vi "main.vi"() -> ()   [LabVIEW 2016]
uses:
  Control 1.ctl
  Antenna.ctl
  Cable 1.ctl
  Cable 2.ctl
  Cable 3.ctl
  Attenuator.ctl
  Amplifier.ctl
  Limit.ctl
  Prescan Spec An Setting.ctl
  Frequency Range.ctl
panel:
  in  "Main":T1(tab)
  in  "Test Configuration":T2(tab)
  in  "Antenna":T3
  in  "Cable 1":T4
  in  "Cable 2":T5
  in  "Cable 3":T6
  in  "Amplifier":T7=enum."10K-2GHz ME813"
  in  "Attenuator":T8
  in  "Limit":T9
  in  "Start Frequecny (MHz)":dbl
  in  "Stop Frequecny (MHz)":dbl
  in  "Generate":bool
  in  "Frequency \nRange":T10
  in  "Prescan \nSpec An \nSetting":T11={"Reference Level (dBuV)"=107.0, "Attenuation (dB)"=10.0, "Step Size (KHz)"=90.0, "RBW (KHz)"=120.0, "VBW (KHz)"=300.0, "Dwell Time (ms)"=0.1, "Detector"=enum."Peak"}
  out "Table Control":string[][](table)
  in  "Prescan Accept":bool
  in  "Start Prescan":bool
  out "Prescan Plot":cluster{"xi used":dbl[], "yi":dbl[]}[](graph)
  in  "Final Accept":bool
  in  "Final Measurement":bool
  out "Equipment ID":string
  in  "VISA input":refnum<visa-resource-name>
  out "Current status":T12
  in  "Stop":bool
  in  "Generate Report":bool
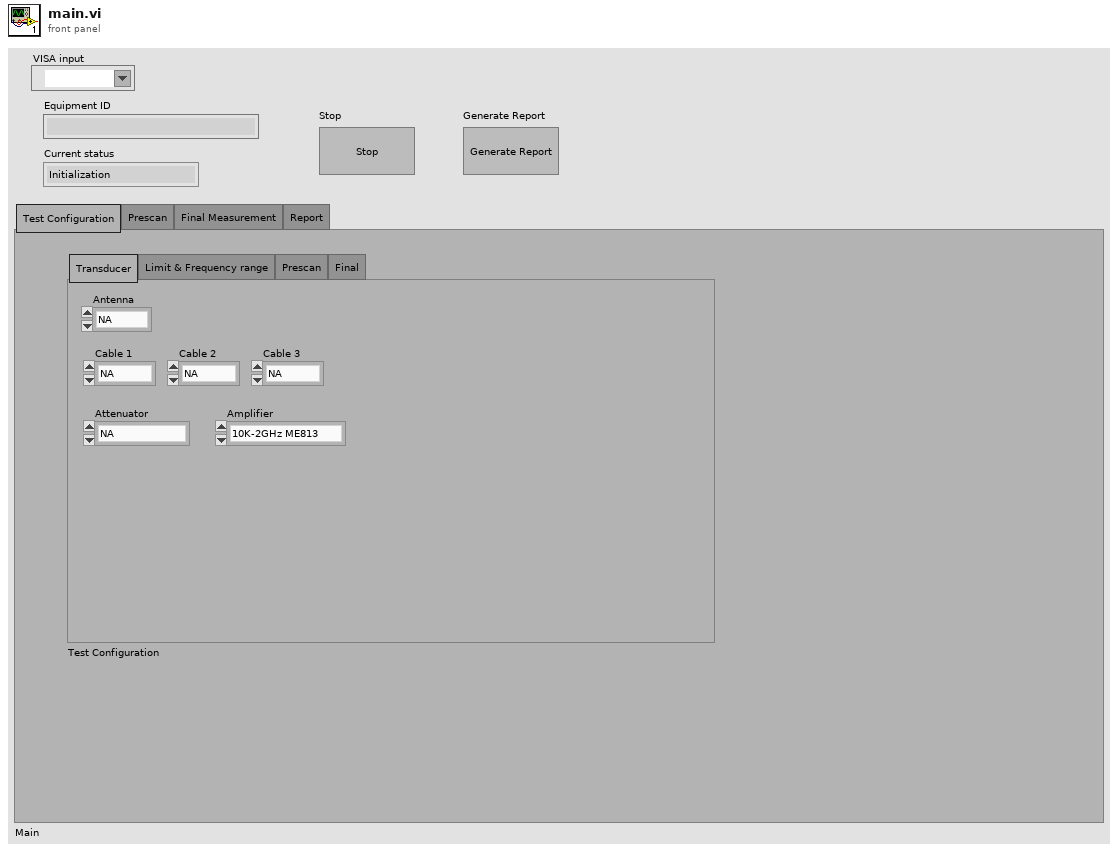
[diagram p1: front panel]
types:
  T1 = enum32{"Test Configuration", "Prescan", "Final Measurement", "Report"}
  T2 = enum32{"Transducer", "Limit & Frequency range", "Prescan", "Final"}
  T3 = typedef "Antenna.ctl" = enum16{"NA", "ME828 Biconical", "ME1284 Periodical"}
  T4 = typedef "Cable 1.ctl" = enum16{"NA", "ME1244", "ME1245", "ME1249"}
  T5 = typedef "Cable 2.ctl" = enum16{"NA", "ME1244", "ME1245", "ME1249"}
  T6 = typedef "Cable 3.ctl" = enum16{"NA", "ME1244", "ME1245", "ME1249"}
  T7 = typedef "Amplifier.ctl" = enum16{"NA", "10K-2GHz ME813", "500M-18GHz ME1241"}
  T8 = typedef "Attenuator.ctl" = enum16{"NA", "6dB-ME811"}
  T9 = typedef "Limit.ctl" = enum16{"NA", "CISPR32 ClassB @ 3m"}
  T10 = typedef "Frequency Range.ctl" = enum32{"20-300MHz", "300-1000MHz", "1-18GHz"}
  T11 = typedef "Prescan Spec An Setting.ctl" = cluster{"Reference Level (dBuV)":dbl, "Attenuation (dB)":dbl, "Step Size (KHz)":dbl, "RBW (KHz)":dbl, "VBW (KHz)":dbl, "Dwell Time (ms)":dbl, "Detector":enum16{"Peak", "CISPR Peak", "Mil Peak", "Quasi Peak", "Average"}}
  T12 = typedef "Control 1.ctl" = enum16{"Initialization", "IDLE (wait for event)", "Prescan test configuration", "Prescan", "Final test configuration", "Final measurement", "Report", "Stop"}
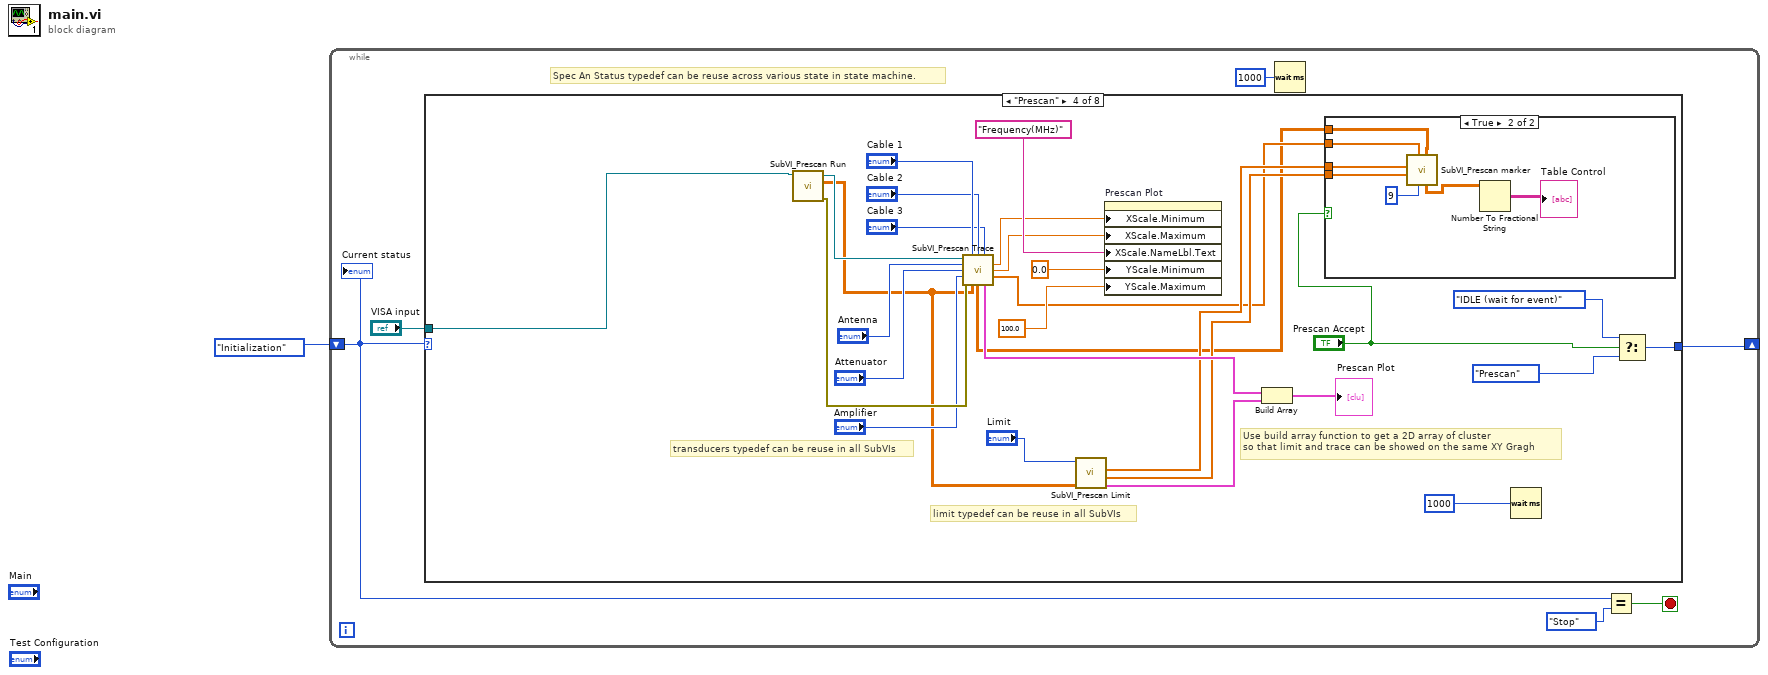
[diagram p0: block diagram]
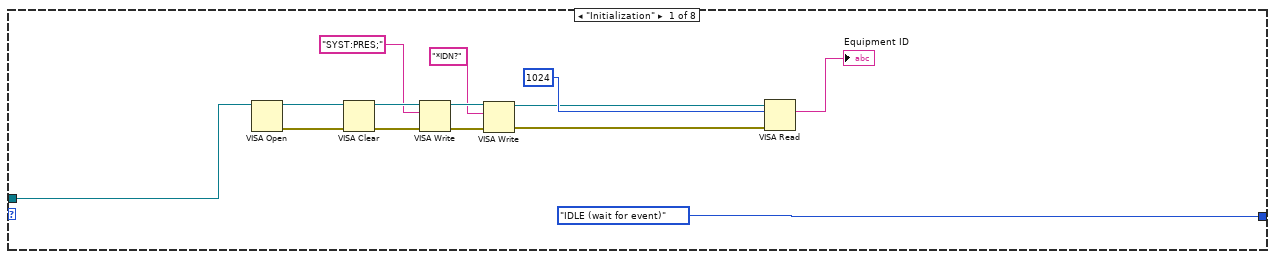
[diagram p2: hidden frame]
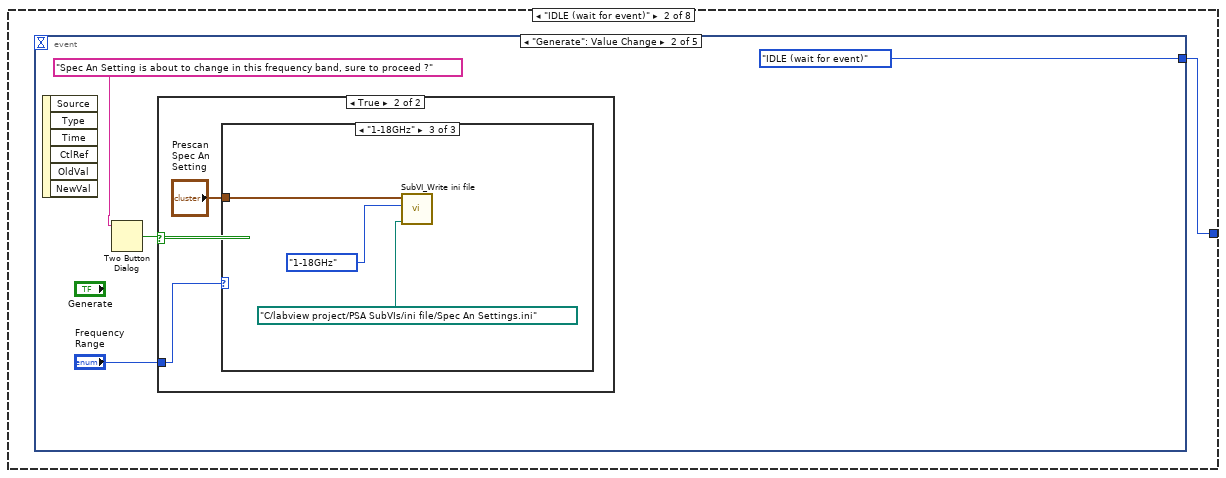
[diagram p3: hidden frame]
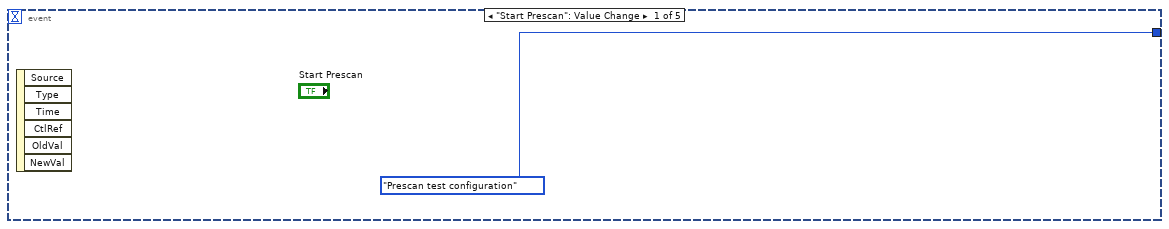
[diagram p4: hidden frame]
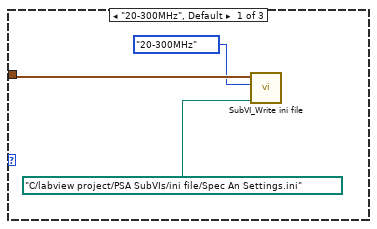
[diagram p6: hidden frame]
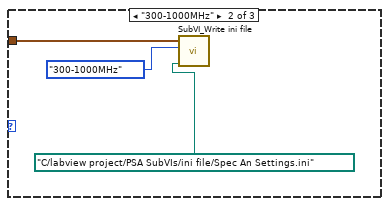
[diagram p7: hidden frame]
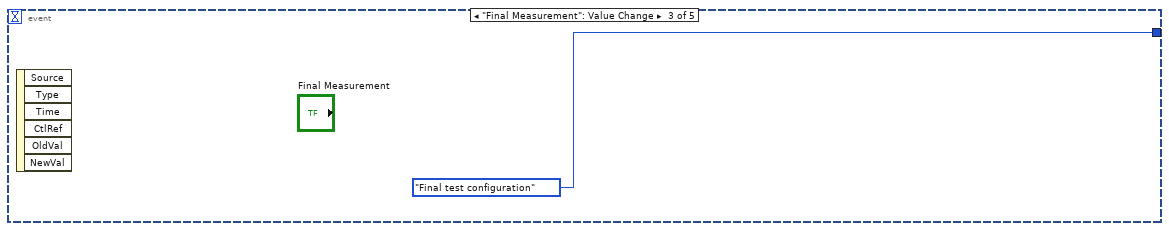
[diagram p8: hidden frame]
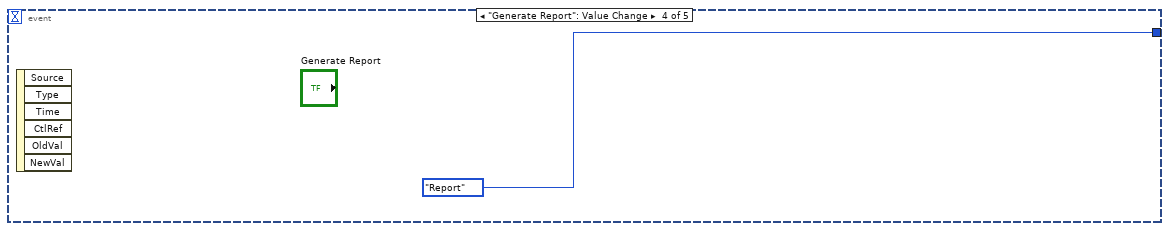
[diagram p9: hidden frame]
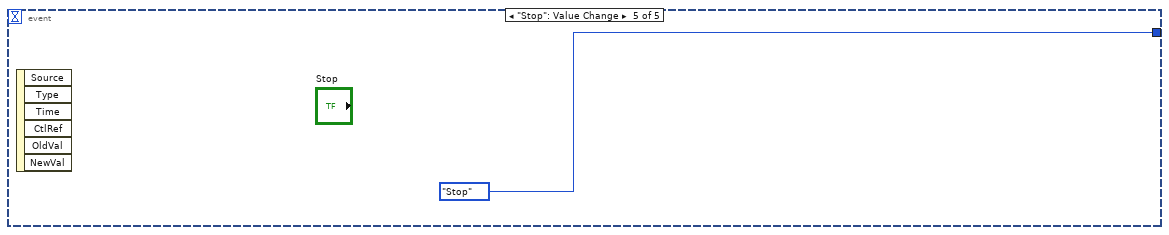
[diagram p10: hidden frame]
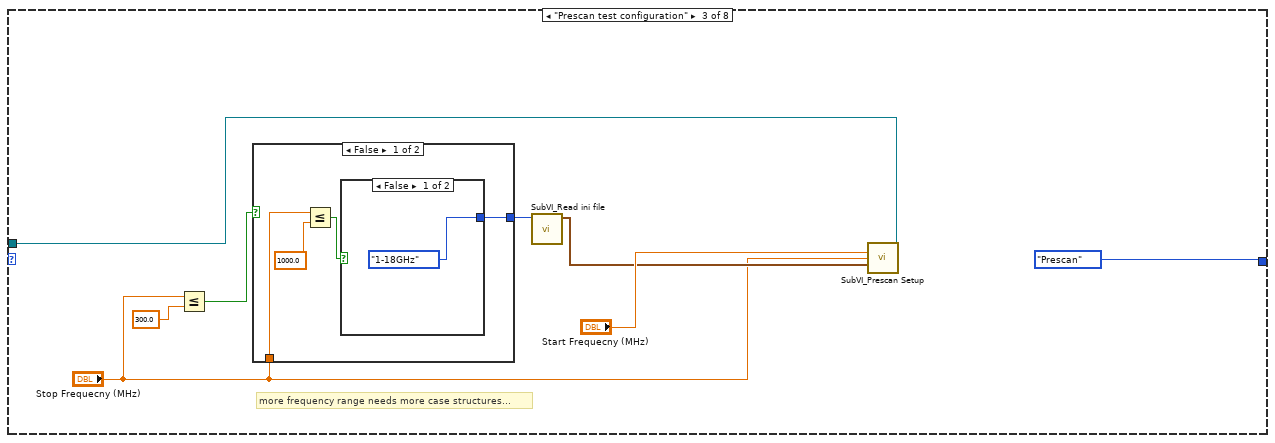
[diagram p11: hidden frame]
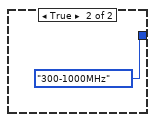
[diagram p12: hidden frame]
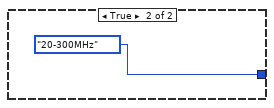
[diagram p13: hidden frame]
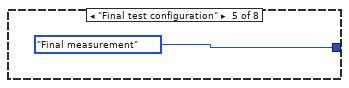
[diagram p15: hidden frame]
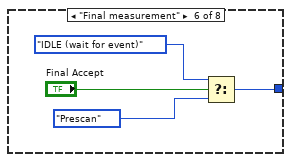
[diagram p16: hidden frame]
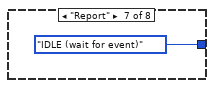
[diagram p17: hidden frame]
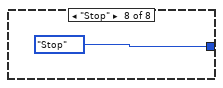
[diagram p18: hidden frame]
diagram:
  n1 = while {
    shift-right: [w6] -> _
    shift-left: Control_1."Initialization" -> [w2]
    stop <- w4 stop-if-true
    # "Spec An Status typedef can be reuse across various state in state machine."
    n2 = case shown="\"Prescan\"" w2 {
      tunnel: [Control_1."IDLE (wait for event)" w22 Control_1."Prescan" w82 Control_1."Final measurement" w93 Control_1."IDLE (wait for event)" Control_1."Stop"] -> w6
      tunnel: "VISA input" -> [w20 _ w47 w81 _ _ _ _]
      frame "Initialization" {
        n3 = VISA Open(VISA resource name=w20) -> (VISA resource name=w19:refnum<visa-resource-name>, error out=w17:errorcluster)  [unwired: 4 in]
        n4 = VISA Clear(VISA resource name=w19, error in (no error)=w17) -> (VISA resource name out=w18:refnum<visa-resource-name>, error out=w16:errorcluster)
        n5 = VISA Write(VISA resource name=w18, write buffer="SYST:PRES;", error in (no error)=w16) -> (VISA resource name out=w12:refnum<visa-resource-name>, error out=w11:errorcluster)  [unwired: 1 out]
        n6 = VISA Write(VISA resource name=w12, write buffer="*IDN?", error in (no error)=w11) -> (VISA resource name out=w9:refnum<visa-resource-name>, error out=w10:errorcluster)  [unwired: 1 out]
        n7 = VISA Read(VISA resource name=w9, byte count=u32 1024, error in (no error)=w10) -> (read buffer=→"Equipment ID":string)  [unwired: 3 out]
      }
      frame "IDLE (wait for event)" {
        n8 = event shown="[1] \"Generate\": Value Change" {
          selector: _ -> [_ _ _ _ _]
          dyn-events: _ -> [_ _ _ _ _]
          timeout: _ -> [_ _ _ _ _]
          tunnel: [Control_1."Prescan test configuration" Control_1."IDLE (wait for event)" Control_1."Final test configuration" Control_1."Report" Control_1."Stop"] -> w22
          event "Start Prescan": Value Change {
            n9 = event-data() -> ()  [unwired: 1 in, 6 out]
          }
          event "Generate": Value Change {
            n10 = event-data() -> ()  [unwired: 1 in, 6 out]
            n11 = Two Button Dialog(message="Spec An Setting is about to change in this frequency band, sure to proceed ?") -> (T button?=w25:bool)  [unwired: 2 in]
            n12 = case shown="True" w25 {
              tunnel: "Frequency \nRange" -> [_ w28]
              frame False {
              }
              frame True {
                n13 = case shown="\"1-18GHz\"" w28 {
                  tunnel: "Prescan \nSpec An \nSetting" -> [w32 w35 w37]
                  frame "20-300MHz", Default {
                    n14 = call "SubVI_Write ini file.vi"("Path"=path "C:/labview project/PSA SubVIs/ini file/Spec An Settings.ini", "Frequency Range"=Frequency_Range."20-300MHz", "Prescan Spec An Setting"=w32) -> ()  [unwired: 9 in]
                  }
                  frame "300-1000MHz" {
                    n15 = call "SubVI_Write ini file.vi"("Path"=path "C:/labview project/PSA SubVIs/ini file/Spec An Settings.ini", "Frequency Range"=Frequency_Range."300-1000MHz", "Prescan Spec An Setting"=w35) -> ()  [unwired: 9 in]
                  }
                  frame "1-18GHz" {
                    n16 = call "SubVI_Write ini file.vi"("Path"=path "C:/labview project/PSA SubVIs/ini file/Spec An Settings.ini", "Frequency Range"=Frequency_Range."1-18GHz", "Prescan Spec An Setting"=w37) -> ()  [unwired: 9 in]
                  }
                }
              }
            }
          }
          event "Final Measurement": Value Change {
            n17 = event-data() -> ()  [unwired: 1 in, 6 out]
          }
          event "Generate Report": Value Change {
            n18 = event-data() -> ()  [unwired: 1 in, 6 out]
          }
          event "Stop": Value Change {
            n19 = event-data() -> ()  [unwired: 1 in, 6 out]
          }
        }
      }
      frame "Prescan test configuration" {
        # "more frequency range needs more case structures..."
        n20 = Less Or Equal?(x="Stop Frequecny (MHz)", y=300.0) -> (x <= y?=w44:bool)
        n21 = case shown="False" w44 {
          tunnel: [w50 Frequency_Range."20-300MHz" ("Frequency Range")] -> w43
          tunnel: "Stop Frequecny (MHz)" -> [w53 _]
          frame False {
            n22 = Less Or Equal?(x=w53, y=1000.0) -> (x <= y?=w51:bool)
            n23 = case shown="False" w51 {
              tunnel: [Frequency_Range."1-18GHz" ("Frequency Range") Frequency_Range."300-1000MHz" ("Frequency Range")] -> w50
              frame False {
              }
              frame True {
              }
            }
          }
          frame True {
          }
        }
        n24 = call "SubVI_Read ini file.vi"("Frequency Range"=w43) -> ("Prescan Spec An \nSetting"=w46:T11)  [unwired: 10 in]
        n25 = call "SubVI_Prescan Setup.vi"("VISA  in"=w47, "Start F (MHz)"="Start Frequecny (MHz)", "Stop F (MHz)"="Stop Frequecny (MHz)", "Prescan Spec An \nSetting"=w46) -> ()  [unwired: 9 in, 3 out]
      }
      frame "Prescan" {
        # "limit typedef can be reuse in all SubVIs"
        # "transducers typedef can be reuse in all SubVIs"
        # "Use build array function to get a 2D array of cluster\nso that limit and trace can be showed on the same XY Gragh"
        n26 = call "SubVI_Prescan Run.vi"("VISA in"=w81) -> ("error out"=w77:errorcluster, "Frequency VS Amplitude (2D array)"=w65:dbl[][], "VISA out"=w76:refnum<visa-resource-name>)  [unwired: 7 in, 1 out]
        n27 = call "SubVI_Prescan Trace.vi"("VISA in"=w76, "Cable 1"="Cable 1", "Cable 2"="Cable 2", "Cable 3"="Cable 3", "Antenna"="Antenna", "Attenuator"="Attenuator", "Amplifier"="Amplifier", "error in (no error)"=w77, "Trace 2D array input"=w65) -> ("Start Frequency"=w78:dbl, "Stop Frequency"=w79:dbl, "Corrected amplitude 1D array"=w59:dbl[], "Completed Result Table"=w57:dbl[][], "Corrected System Trace"=w64:cluster{dbl[], "x+y":dbl[]})  [unwired: 2 out]
        n28 = call "SubVI_Prescan Limit.vi"("Input trace 2D array"=w65, "Limit"="Limit") -> ("Output Limit Cluster"=w63:cluster{"xi used":dbl[], "yi":dbl[]}, "limit 1D array"=w60:dbl[], "frequency 1D array"=w61:dbl[])  [unwired: 6 in, 1 out]
        n29 = property on="Prescan Plot" class="XYGraph (strict)"("XScale.Minimum"=w78, "XScale.Maximum"=w79, "XScale.NameLbl.Text"="Frequency(MHz)" ("X Scale.Name Label.Text"), "YScale.Minimum"=0.0 ("Y Scale.Range:Minimum"), "YScale.Maximum"=100.0 ("Y Scale.Range:Maximum")) -> ()  [unwired: 2 in, 2 out]
        n30 = Build Array(w64, w63) -> (→"Prescan Plot":cluster{"xi used":dbl[], "yi":dbl[]}[])
        n31 = case shown="True" "Prescan Accept" {
          tunnel: w61 -> [_ w91]
          tunnel: w60 -> [_ w90]
          tunnel: w59 -> [_ w89]
          tunnel: w57 -> [_ w88]
          frame False {
          }
          frame True {
            n32 = call "SubVI_Prescan marker.vi"("corrected 2D array"=w88, "Column to Sort on"=9, "corrected amplitude 1D arrray"=w89, "limit 1D array"=w90, "frequency 1D array"=w91) -> ("6 entries in table"=w86:dbl[][])  [unwired: 4 in, 2 out]
            n33 = Number To Fractional String(number=w86) -> (F-format string=→"Table Control":string[][])  [unwired: 3 in]
          }
        }
        n34 = Wait (ms)(milliseconds to wait=u32 1000) -> ()  [unwired: 1 out]
        n35 = Select(t=Control_1."IDLE (wait for event)", s="Prescan Accept", f=Control_1."Prescan") -> (s? t:f=w82:T12)
      }
      frame "Final test configuration" {
      }
      frame "Final measurement" {
        n36 = Select(t=Control_1."IDLE (wait for event)", s="Final Accept", f=Control_1."Prescan") -> (s? t:f=w93:T12)
      }
      frame "Report" {
      }
      frame "Stop" {
      }
    }
    n37 = Wait (ms)(milliseconds to wait=u32 1000) -> ()  [unwired: 1 out]
    n38 = Equal?(x=w2, y=Control_1."Stop") -> (x = y?=w4:bool)
    "Current status" <- w2
  }
